vi "LS218_CHECK_CONFIG.vi"(8 "Type sondes 5-8":u16, 9 "Type sondes 1-4":u16, 10 "table_voies":T1(array[cluster])) -> (0 "INTYPE=diode":bool[](array[boolean]), 1 "conf_check":bool[](array[boolean]), 2 "INCRV=diode":bool[](array[boolean]), 3 "conf_OK":bool)   [LabVIEW 2016]
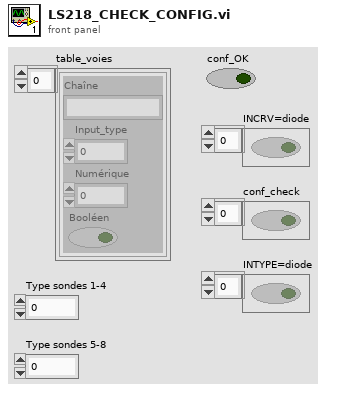
[diagram p1: front panel]
types:
  T1 = cluster{"Chaîne":string, "Input_type":u16, "Numérique":dbl, "Booléen":bool}[]
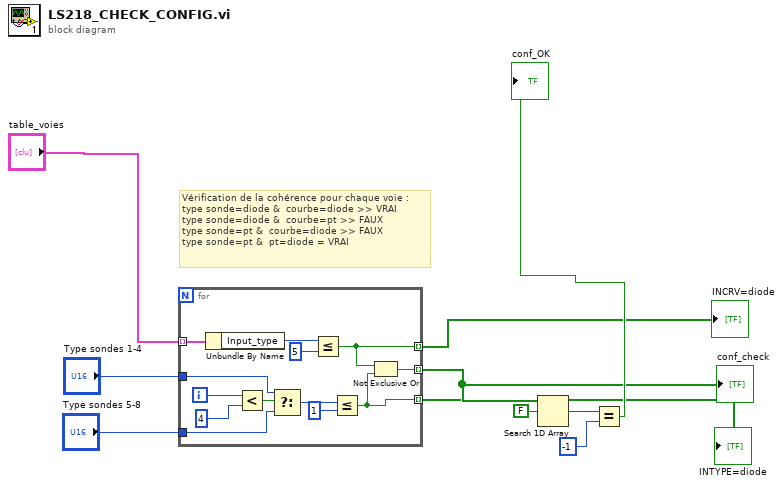
[diagram p0: block diagram]
diagram:
  # "Vérification de la cohérence pour chaque voie : \ntype sonde=diode &  courbe=diode >> VRAI\ntype sonde=diode &  courbe=pt >> FAUX\ntype sonde=pt &  courbe=diode >> FAUX\ntype sonde=pt &  pt=diode = VRAI"
  n1 = for {
    tunnel: "table_voies" -> [w23] mode=indexing
    tunnel: "Type sondes 1-4" -> [w19]
    tunnel: "Type sondes 5-8" -> [w18]
    tunnel: [w13] -> w3 mode=indexing
    tunnel: [w12] -> w4 mode=indexing
    tunnel: [w11] -> w6 mode=indexing
    i -> [w22]
    n2 = Unbundle By Name(w23) -> ("Input_type"=w17:u16)
    n3 = Less?(x=w22, y=4) -> (x < y?=w20:bool)
    n4 = Select(t=w19, s=w20, f=w18) -> (s? t:f=w15:u16)
    n5 = Less Or Equal?(x=w17, y=u16 5) -> (x <= y?=w13:bool)
    n6 = Less Or Equal?(x=w15, y=u16 1) -> (x <= y?=w12:bool)
    n7 = Not Exclusive Or(1:w12, 2:w13) -> (0:w11:bool)
  }
  "conf_check" <- w6
  "INTYPE=diode" <- w4
  "INCRV=diode" <- w3
  n8 = Search 1D Array(1D array=w6, element=FALSE ("élément")) -> (index of element=w8:i32)  [unwired: 1 in]
  n9 = Equal?(x=w8, y=-1) -> (x = y?=→"conf_OK":bool)
